vi "switch off request.vi"(8 "Z4(AutoSetState)":T1(array[ring])=[enum."stop ready", enum."stop ready", enum."stop ready", enum."stop ready"], 9 "Z4_tmp(AutoSetState)":T1(array[ring])=[enum."stop ready", enum."stop ready", enum."stop ready", enum."stop ready"], 10 "Z3(State)":T1(array[ring])=[enum."stop ready", enum."stop ready", enum."stop ready", enum."stop ready"], 11 "Z1(CmdSource)":T2(array[ring])=[enum."auto", enum."auto", enum."auto", enum."auto"]) -> (1 "N":i32, 2 "ok":bool, 3 "Z4_out(AutoSetState)":T1(array[ring])=[enum."stop ready", enum."stop ready", enum."stop ready", enum."stop ready"])   [LabVIEW 2019, in "Userlib.lvlib"]
uses:
  Userlib.lvlib
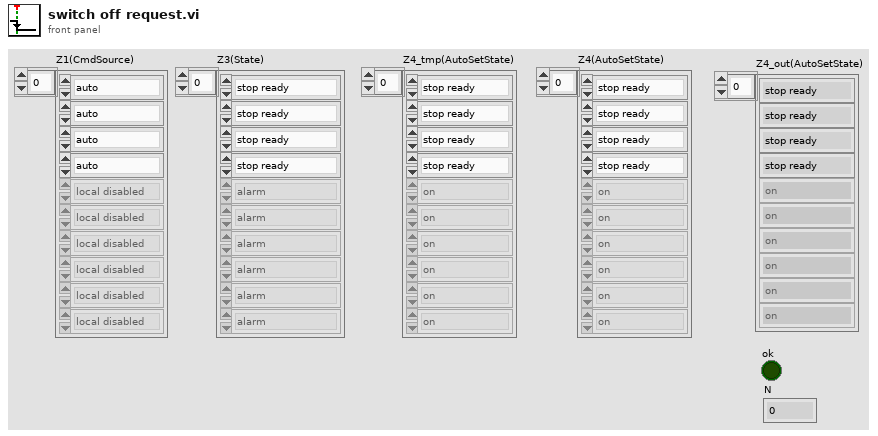
[diagram p1: front panel]
types:
  T1 = enum32{"alarm", "disabled", "not ready", "stop ready", "reserv", "switched off", "switched on", "check", "on min", "decrease speed", "on", "increase speed", "on max"}[]
  T2 = enum32{"local disabled", "local hand", "hand", "auto", "dist"}[]
  T3 = enum32{"alarm", "disabled", "not ready", "stop ready", "reserv", "switched off", "switched on", "check", "on min", "decrease speed", "on", "increase speed", "on max"}
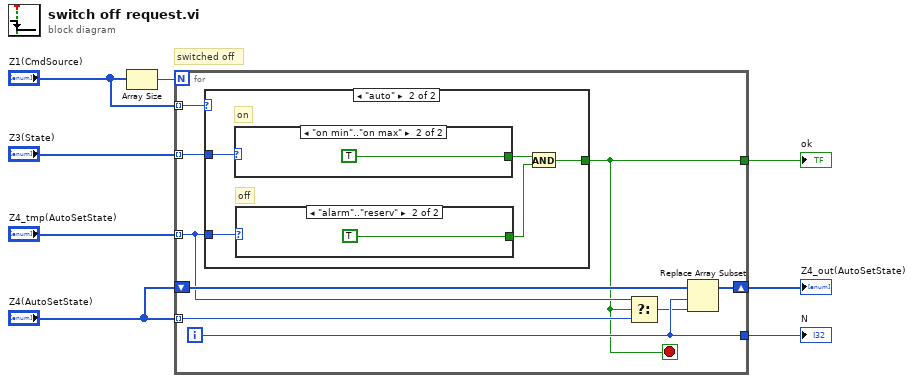
[diagram p0: block diagram]
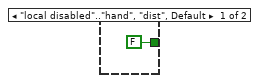
[diagram p2: hidden frame]
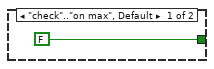
[diagram p3: hidden frame]
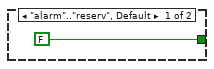
[diagram p4: hidden frame]
diagram:
  # "switched off"
  n1 = Array Size(array="Z1(CmdSource)") -> (size(s)=w6:i32)
  n2 = for {
    N: w6 -> [_]
    tunnel: "Z3(State)" -> [w12] mode=indexing
    tunnel: "Z1(CmdSource)" -> [w11] mode=indexing
    tunnel: [w15] -> w4
    tunnel: "Z4_tmp(AutoSetState)" -> [w10] mode=indexing
    tunnel: [w9] -> w3
    tunnel: "Z4(AutoSetState)" -> [w17] mode=indexing
    shift-right: [w13] -> w2
    shift-left: "Z4(AutoSetState)" -> [w16]
    i -> [w15]
    stop <- w9 stop-if-true
    n3 = case shown="\"auto\"" w11 {
      tunnel: w12 -> [_ w22]
      tunnel: w10 -> [_ w21]
      tunnel: [FALSE w23] -> w9
      frame "local disabled".."hand", "dist", Default {
      }
      frame "auto" {
        # "off"
        # "on"
        n4 = case shown="\"on min\"..\"on max\"" w22 {
          tunnel: [FALSE TRUE] -> w20
          frame "alarm".."reserv", Default {
          }
          frame "on min".."on max" {
          }
        }
        n5 = case shown="\"alarm\"..\"reserv\"" w21 {
          tunnel: [FALSE TRUE] -> w19
          frame "check".."on max", Default {
          }
          frame "alarm".."reserv" {
          }
        }
        n6 = And(x=w20, y=w19) -> (x .and. y?=w23:bool)
      }
    }
    n7 = Select(t=w10, s=w9, f=w17) -> (s? t:f=w14:T3)
    n8 = Replace Array Subset(array=w16, new element=w14, index=w15) -> (w13:T1)
  }
  "Z4_out(AutoSetState)" <- w2
  "N" <- w4
  "ok" <- w3
